vi "MTMount_putSample_AuxliaryCabinetAzimuth.vi"(8 "error in (no error)":errorcluster, 11 "Auxliary_Cabinet_Azimuth_Ctl":T1) -> (0 "error out":errorcluster, 2 "function return":i32, 3 "Auxliary_Cabinet_Azimuth_Ctl out":T1)   [LabVIEW 2018, in "SALLV_MTMount.lvlib"]
doc: "int MTMount_shm_putSample_Auxliary_Cabinet_AzimuthLV(MTMount_Auxliary_Cabinet_AzimuthLV *Auxliary_Cabinet_Azimuth_Ctl );"
uses:
  SALLV_MTMount.lvlib
  DataTypes/Auxliary_Cabinet_Azimuth.ctl
  SALLV_MTMount.so
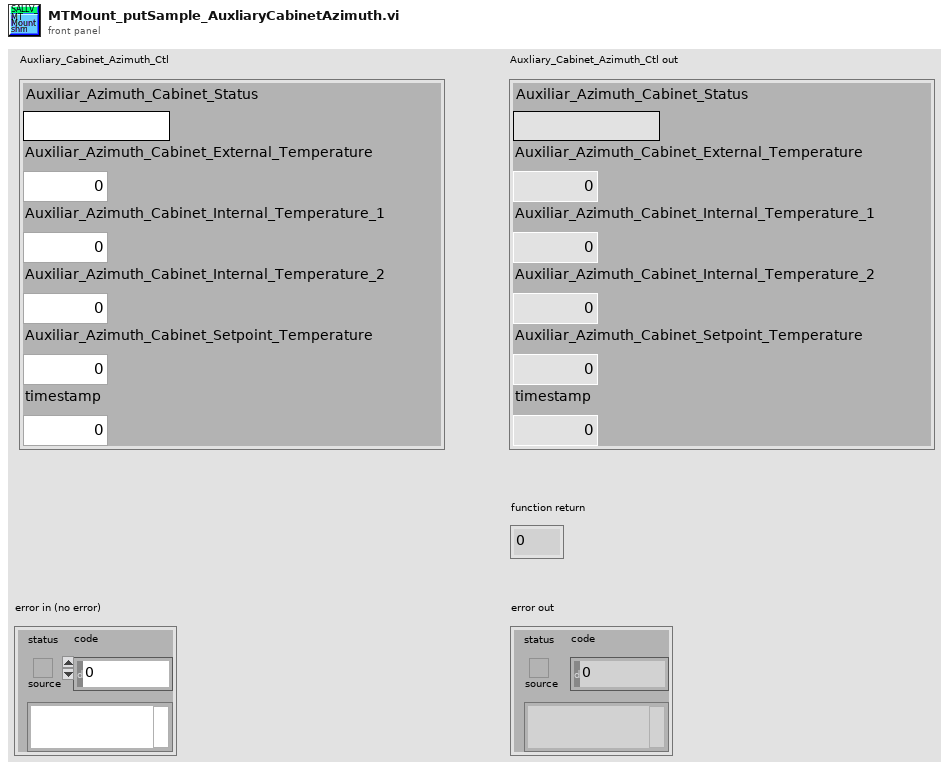
[diagram p1: front panel]
types:
  T1 = typedef "SALLV_MTMount.lvlib/Auxliary_Cabinet_Azimuth.ctl" = cluster{"Auxiliar_Azimuth_Cabinet_Status":string, "Auxiliar_Azimuth_Cabinet_External_Temperature":dbl, "Auxiliar_Azimuth_Cabinet_Internal_Temperature_1":dbl, "Auxiliar_Azimuth_Cabinet_Internal_Temperature_2":dbl, "Auxiliar_Azimuth_Cabinet_Setpoint_Temperature":dbl, "timestamp":dbl}
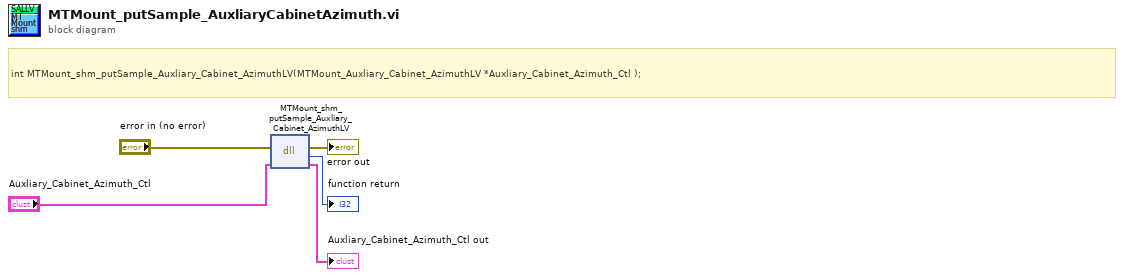
[diagram p0: block diagram]
diagram:
  # "int MTMount_shm_putSample_Auxliary_Cabinet_AzimuthLV(MTMount_Auxliary_Cabinet_AzimuthLV *Auxliary_Cabinet_Azimuth_Ctl );"
  n1 = dll-call lib="home/ttsai/Document/salApiMTMount/SALLV_MTMount/SALLV_MTMount.*" fn="MTMount_shm_putSample_Auxliary_Cabinet_AzimuthLV"(error in="error in (no error)", "Auxliary_Cabinet_Azimuth_Ctl"="Auxliary_Cabinet_Azimuth_Ctl") -> (error out=→"error out":errorcluster, →"function return":i32, "Auxliary_Cabinet_Azimuth_Ctl"=→"Auxliary_Cabinet_Azimuth_Ctl out":T1)  [unwired: 2 in, 1 out]
